vi "MGI Find 2D Intersection of 2 Lines.vi"(8 "error in (no error)":errorcluster, 10 "Line 2[start, end][x,y]":dbl[][](array[numeric]) format="%#.15f", 11 "Line 1[start, end][x,y]":dbl[][](array[numeric])) -> (0 "error out":errorcluster, 1 "Intersection within Line2 Segment?":bool, 2 "Intersection within Line1 Segment?":bool, 3 "Intersection[x,y]":dbl[](array[numeric]) format="%#_12g")   [LabVIEW 2016]
doc: "Finds the intersection of 2 lines. If the lines are parallel, then an argument error (code 1) is output.\nThe lines are specified using 2 points for each line. The points are specified as rows in a 2D array where the first column is x and the second is y.\n\nAuthored by Shawn D. Walpole\nsupport@mooregoodideas.com\nwww.mooregoodideas.com\n\nCopyright (c) 2010, Moore Good Ideas, Inc.\n\nAll rights reserved.\n\nRedistribution and use in source and binary forms, with or without modification, are permitted provided that the following conditions are met:\n\n * Redistributions of source code must retain the above copyright notice, this list of conditions and the following disclaimer.\n * Redistributions in binary form must reproduce the above copyright notice, this list of conditions and the following disclaimer in the documentation and/or other materials provided with the distribution.\n * Neither the name of Moore Good Ideas, Inc. nor the names of its contributors may be used to endorse or promote products derived from this software without specific prior written permission.\n\nTHIS SOFTWARE IS PROVIDED BY THE COPYRIGHT HOLDERS AND CONTRIBUTORS \"AS IS\" AND ANY EXPRESS OR IMPLIED WARRANTIES, INCLUDING, BUT NOT LIMITED TO, THE IMPLIED WARRANTIES OF MERCHANTABILITY AND FITNESS FOR A PARTICULAR PURPOSE ARE DISCLAIMED. IN NO EVENT SHALL THE COPYRIGHT OWNER OR CONTRIBUTORS BE LIABLE FOR ANY DIRECT, INDIRECT, INCIDENTAL, SPECIAL, EXEMPLARY, OR CONSEQUENTIAL DAMAGES (INCLUDING, BUT NOT LIMITED TO, PROCUREMENT OF SUBSTITUTE GOODS OR SERVICES; LOSS OF USE, DATA, OR PROFITS; OR BUSINESS INTERRUPTION) HOWEVER CAUSED AND ON ANY THEORY OF LIABILITY, WHETHER IN CONTRACT, STRICT LIABILITY, OR TORT (INCLUDING NEGLIGENCE OR OTHERWISE) ARISING IN ANY WAY OUT OF THE USE OF THIS SOFTWARE, EVEN IF ADVISED OF THE POSSIBILITY OF SUCH DAMAGE."
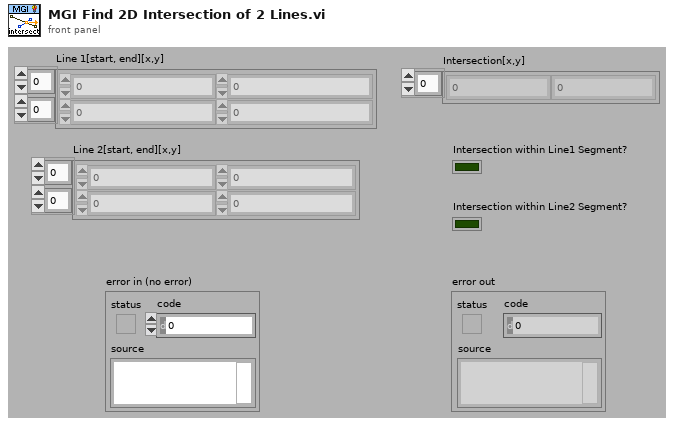
[diagram p1: front panel]
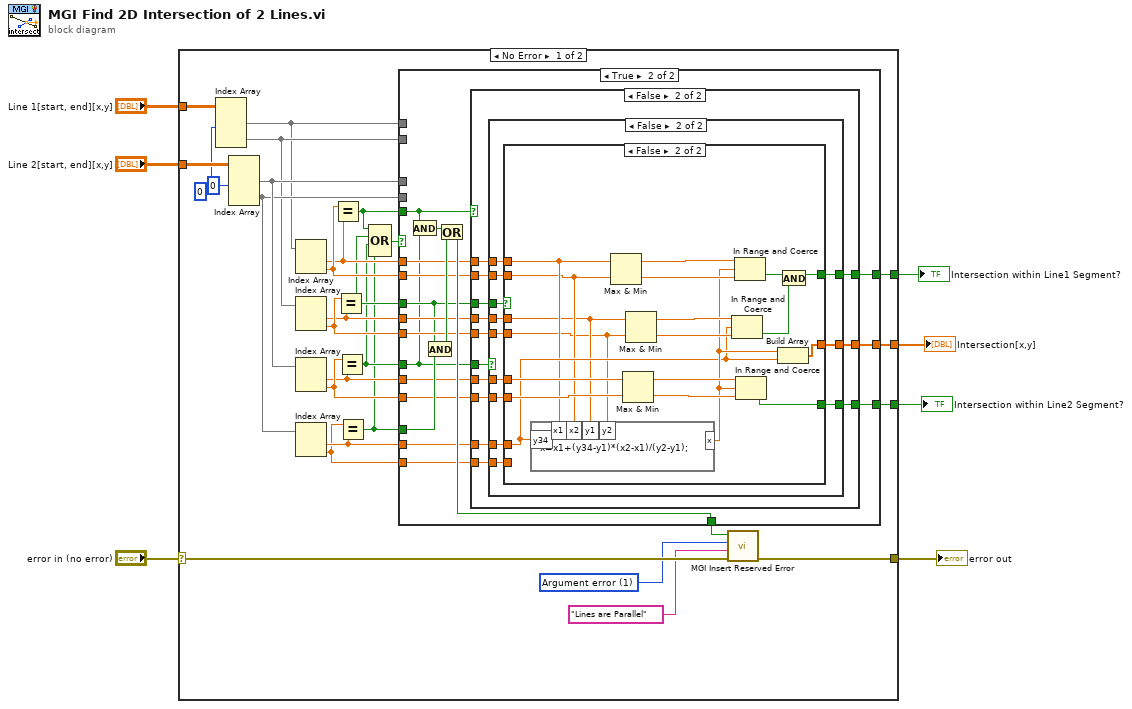
[diagram p0: block diagram]
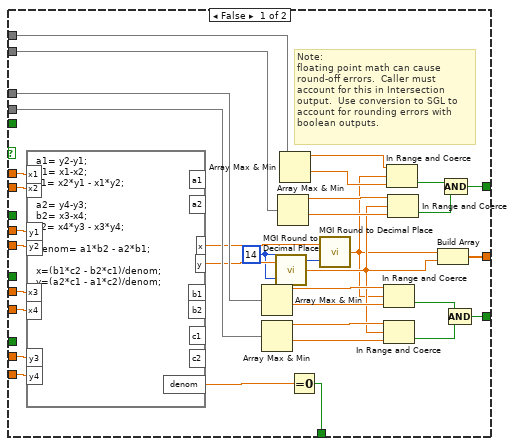
[diagram p2: hidden frame]
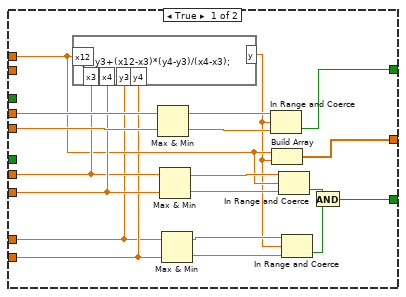
[diagram p3: hidden frame]
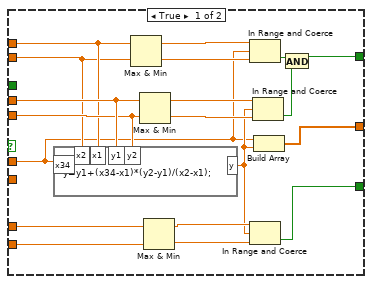
[diagram p4: hidden frame]
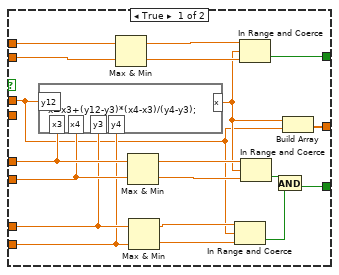
[diagram p5: hidden frame]
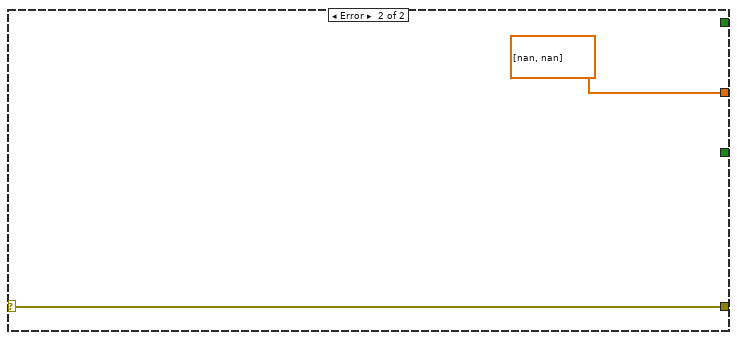
[diagram p6: hidden frame]
diagram:
  n1 = case shown="No Error" "error in (no error)" {
    selector: "error in (no error)" -> [w35 w191]
    tunnel: [w34 w191] -> w6
    tunnel: "Line 1[start, end][x,y]" -> [w30 _]
    tunnel: "Line 2[start, end][x,y]" -> [w29 _]
    tunnel: [w36 dbl[] [nan, nan]] -> w3
    tunnel: [w28 _] -> w2
    tunnel: [w27 _] -> w1
    frame No Error {
      w32 = u16 1 items=["No error", "Argument error", "Memory is full", "Out of zone", "End of file", "File already open", "Generic file I/O error", "File not found", "File permission error", "Disk is full", "Duplicate path", "Too many files open", "System feature not enabled", "Resource file not found", "Cannot add resource", "Resource not found", "Image not found", "Image memory error", "Pen does not exist", "Config type invalid", "Config token not found", "Config parse error", "Config memory error", "Bad external code format", "Bad external code offset", "External code not present", "Null window", "Destroy window error", "Null menu", "Print aborted", "Bad print record", "Print driver error", "Windows error during printing", "Memory error during printing", "Print dialog error", "Generic print error", "Invalid device refnum", "Device not found", "Device parameter error", "Device unit error", "Cannot open device", "Device call aborted", "Generic error", "Cancelled by user", "Object ID too low", "Object ID too high", "Object not in heap", "Unknown heap", "Unknown object (invalid DefProc)", "Unknown object (DefProc not in table)", "Message out of range", "Invalid (null) method", "Unknown message", "Manager call not supported", "Bad address", "Network operation in progress", "Network operation timed out", "Connection is busy", "Network attribute not supported", "Network error", "Address in use", "System out of memory", "Connection aborted", "Connection refused", "Not connected", "Already connected", "Connection closed", "Initialization error (interapplication manager)", "Bad occurrence", "Wait on unbound occurrence handler", "Occurrence queue overflow", "Datalog type conflict", "Unused", "Unrecognized type (interapplication manager)", "Memory corrupt", "Failed to make temporary DLL", "Old CIN version", "Drag socket not found", "Failed to load drop-object", "Failed to register OLE object", "Failed to release OLE object", "Format specifier type mismatch", "Unknown format specifier", "Too few format specifiers", "Too many format specifiers", "Scan failed", "Newer CIN version", "OLE Convert", "Runtime menu error", "Password tampered", "Unknown error code"] ("Reserved Error Code (Generic error)")
      n2 = Index Array(array=w30, index (col) #1=0 ("disabled index (col)")) -> (element #1=w21:dbl[], element #2=w22:dbl[])  [unwired: 3 in]
      n3 = Index Array(array=w29, index (col) #1=0 ("disabled index (col)")) -> (element #1=w24:dbl[], element #2=w23:dbl[])  [unwired: 3 in]
      n4 = Index Array(array=w21) -> (element #1=w19:dbl, element #2=w20:dbl)  [unwired: 2 in]
      n5 = Index Array(array=w22) -> (element #1=w17:dbl, element #2=w18:dbl)  [unwired: 2 in]
      n6 = Index Array(array=w24) -> (element #1=w15:dbl, element #2=w16:dbl)  [unwired: 2 in]
      n7 = Index Array(array=w23) -> (element #1=w14:dbl, element #2=w13:dbl)  [unwired: 2 in]
      n8 = Equal?(x=w20, y=w19) -> (x = y?=w11:bool)
      n9 = Equal?(x=w18, y=w17) -> (x = y?=w10:bool)
      n10 = Equal?(x=w16, y=w15) -> (x = y?=w9:bool)
      n11 = Equal?(x=w13, y=w14) -> (x = y?=w8:bool)
      n12 = Compound Arithmetic op=OR(w11, w10, w9, w8) -> (w12:bool)
      n13 = case shown="True" w12 {
        tunnel: [w70 w75] -> w36
        tunnel: [w68 w85] -> w33
        tunnel: [w63 w74] -> w28
        tunnel: [w62 w73] -> w27
        tunnel: w24 -> [w53 _]
        tunnel: w23 -> [w52 _]
        tunnel: w22 -> [w51 _]
        tunnel: w21 -> [w50 _]
        tunnel: w20 -> [w44 w82]
        tunnel: w19 -> [w43 w83]
        tunnel: w18 -> [w42 w80]
        tunnel: w17 -> [w41 w81]
        tunnel: w16 -> [w40 w78]
        tunnel: w15 -> [w39 w79]
        tunnel: w14 -> [w38 w77]
        tunnel: w13 -> [w37 w76]
        tunnel: w11 -> [_ w84]
        tunnel: w10 -> [_ w72]
        tunnel: w9 -> [_ w71]
        tunnel: w8 -> [_ w88]
        frame False {
          w45 = 14 ("Decimal Digits")
          # "Note:\nfloating point math can cause round-off errors.  Caller must account for this in Intersection output.  Use conversion to SGL to account for rounding errors with boolean outputs."
          n14 = formula code="a1= y2-y1;\nb1= x1-x2;\nc1= x2*y1 - x1*y2;\n\na2= y4-y3;\nb2= x3-x4;\nc2= x4*y3 - x3*y4;\n\ndenom= a1*b2 - a2*b1;\n\nx=(b1*c2 - b2*c1)/denom;\ny=(a2*c1 - a1*c2)/denom;"("y2"=w42, "y1"=w41, "x2"=w44, "x1"=w43, "y4"=w37, "y3"=w38, "x4"=w40, "x3"=w39) -> ("denom"=w69:dbl, "x"=w47:dbl, "y"=w49:dbl)  [unwired: 6 out]
          n15 = Array Max & Min(array=w53) -> (max value=w57:dbl, min value=w56:dbl)  [unwired: 2 out]
          n16 = Array Max & Min(array=w52) -> (max value=w55:dbl, min value=w54:dbl)  [unwired: 2 out]
          n17 = call <userlib>:"MGI Round to Decimal Place.vi"("Decimal Digits"=w45, "Number"=w49) -> ("Rounded"=w48:dbl)  [unwired: 1 in]
          n18 = Array Max & Min(array=w51) -> (max value=w59:dbl, min value=w58:dbl)  [unwired: 2 out]
          n19 = Array Max & Min(array=w50) -> (max value=w61:dbl, min value=w60:dbl)  [unwired: 2 out]
          n20 = Equal To 0?(x=w69) -> (x = 0?=w68:bool)
          n21 = call <userlib>:"MGI Round to Decimal Place.vi"("Decimal Digits"=w45, "Number"=w47) -> ("Rounded"=w46:dbl)  [unwired: 1 in]
          n22 = In Range and Coerce(upper limit=w57, x=w46, lower limit=w56) -> (In Range?=w67:bool)  [unwired: 1 out]
          n23 = In Range and Coerce(upper limit=w55, x=w48, lower limit=w54) -> (In Range?=w66:bool)  [unwired: 1 out]
          n24 = In Range and Coerce(upper limit=w61, x=w46, lower limit=w60) -> (In Range?=w65:bool)  [unwired: 1 out]
          n25 = In Range and Coerce(upper limit=w59, x=w48, lower limit=w58) -> (In Range?=w64:bool)  [unwired: 1 out]
          n26 = Build Array(w46, w48) -> (w70:dbl[])
          n27 = Compound Arithmetic op=AND(w65, w64) -> (w63:bool)
          n28 = Compound Arithmetic op=AND(w67, w66) -> (w62:bool)
        }
        frame True {
          n29 = And(x=w84, y=w71) -> (x .and. y?=w86:bool)
          n30 = And(x=w72, y=w88) -> (x .and. y?=w87:bool)
          n31 = Or(x=w86, y=w87) -> (x .or. y?=w85:bool)
          n32 = case shown="False" w84 {
            tunnel: w83 -> [w97 w114]
            tunnel: w82 -> [_ w108]
            tunnel: w81 -> [w104 w117]
            tunnel: w80 -> [w105 w118]
            tunnel: w79 -> [w100 w115]
            tunnel: w78 -> [w101 w116]
            tunnel: w77 -> [w95 w112]
            tunnel: w76 -> [w96 w113]
            tunnel: [w107 w120] -> w75
            tunnel: [w106 w119] -> w74
            tunnel: [w89 w111] -> w73
            tunnel: w72 -> [_ w109]
            tunnel: w71 -> [_ w110]
            frame True {
              n33 = formula code="y=y3+(x12-x3)*(y4-y3)/(x4-x3);"("x12"=w97, "x3"=w100, "x4"=w101, "y3"=w95, "y4"=w96) -> ("y"=w92:dbl)
              n34 = Max & Min(x=w104, y=w105) -> (max(x,y)=w103:dbl, min(x,y)=w102:dbl)
              n35 = Max & Min(x=w100, y=w101) -> (max(x,y)=w99:dbl, min(x,y)=w98:dbl)
              n36 = Max & Min(x=w95, y=w96) -> (max(x,y)=w93:dbl, min(x,y)=w94:dbl)
              n37 = In Range and Coerce(upper limit=w103, x=w92, lower limit=w102) -> (In Range?=w106:bool)  [unwired: 1 out]
              n38 = Build Array(w97, w92) -> (w107:dbl[])
              n39 = In Range and Coerce(upper limit=w99, x=w97, lower limit=w98) -> (In Range?=w90:bool)  [unwired: 1 out]
              n40 = In Range and Coerce(upper limit=w93, x=w92, lower limit=w94) -> (In Range?=w91:bool)  [unwired: 1 out]
              n41 = And(x=w90, y=w91) -> (x .and. y?=w89:bool)
            }
            frame False {
              n42 = case shown="False" w110 {
                tunnel: [w139 w151] -> w120
                tunnel: [w123 w143] -> w119
                tunnel: w118 -> [w127 w147]
                tunnel: w117 -> [w128 w148]
                tunnel: w116 -> [_ w140]
                tunnel: w115 -> [w121 w142]
                tunnel: w114 -> [w125 w145]
                tunnel: w113 -> [w133 w150]
                tunnel: w112 -> [w132 w149]
                tunnel: [w126 w146] -> w111
                tunnel: w109 -> [_ w141]
                tunnel: w108 -> [w124 w144]
                frame True {
                  n43 = formula code="y=y1+(x34-x1)*(y2-y1)/(x2-x1);"("x1"=w125, "x34"=w121, "x2"=w124, "y1"=w128, "y2"=w127) -> ("y"=w129:dbl)
                  n44 = Max & Min(x=w125, y=w124) -> (max(x,y)=w135:dbl, min(x,y)=w134:dbl)
                  n45 = Max & Min(x=w128, y=w127) -> (max(x,y)=w137:dbl, min(x,y)=w136:dbl)
                  n46 = Max & Min(x=w132, y=w133) -> (max(x,y)=w130:dbl, min(x,y)=w131:dbl)
                  n47 = In Range and Coerce(upper limit=w135, x=w121, lower limit=w134) -> (In Range?=w122:bool)  [unwired: 1 out]
                  n48 = In Range and Coerce(upper limit=w130, x=w129, lower limit=w131) -> (In Range?=w126:bool)  [unwired: 1 out]
                  n49 = In Range and Coerce(upper limit=w137, x=w129, lower limit=w136) -> (In Range?=w138:bool)  [unwired: 1 out]
                  n50 = Build Array(w121, w129) -> (w139:dbl[])
                  n51 = And(x=w122, y=w138) -> (x .and. y?=w123:bool)
                }
                frame False {
                  n52 = case shown="False" w141 {
                    tunnel: [w170 w189] -> w151
                    tunnel: w150 -> [w157 _]
                    tunnel: w149 -> [w158 w179]
                    tunnel: w148 -> [w154 w176]
                    tunnel: w147 -> [_ w175]
                    tunnel: [w153 w174] -> w146
                    tunnel: w145 -> [w162 w178]
                    tunnel: w144 -> [w161 w177]
                    tunnel: [w155 w171] -> w143
                    tunnel: w142 -> [w160 w182]
                    tunnel: w140 -> [w159 w181]
                    frame True {
                      n53 = formula code="x=x3+(y12-y3)*(x4-x3)/(y4-y3);"("y3"=w158, "y12"=w154, "y4"=w157, "x3"=w160, "x4"=w159) -> ("x"=w156:dbl)
                      n54 = Max & Min(x=w162, y=w161) -> (max(x,y)=w167:dbl, min(x,y)=w166:dbl)
                      n55 = Max & Min(x=w160, y=w159) -> (max(x,y)=w169:dbl, min(x,y)=w168:dbl)
                      n56 = Max & Min(x=w158, y=w157) -> (max(x,y)=w164:dbl, min(x,y)=w165:dbl)
                      n57 = In Range and Coerce(upper limit=w164, x=w154, lower limit=w165) -> (In Range?=w163:bool)  [unwired: 1 out]
                      n58 = In Range and Coerce(upper limit=w167, x=w156, lower limit=w166) -> (In Range?=w155:bool)  [unwired: 1 out]
                      n59 = In Range and Coerce(upper limit=w169, x=w156, lower limit=w168) -> (In Range?=w152:bool)  [unwired: 1 out]
                      n60 = And(x=w152, y=w163) -> (x .and. y?=w153:bool)
                      n61 = Build Array(w156, w154) -> (w170:dbl[])
                    }
                    frame False {
                      n62 = formula code="x=x1+(y34-y1)*(x2-x1)/(y2-y1);"("y1"=w176, "y34"=w179, "y2"=w175, "x1"=w178, "x2"=w177) -> ("x"=w180:dbl)
                      n63 = Max & Min(x=w178, y=w177) -> (max(x,y)=w186:dbl, min(x,y)=w185:dbl)
                      n64 = Max & Min(x=w182, y=w181) -> (max(x,y)=w188:dbl, min(x,y)=w187:dbl)
                      n65 = Max & Min(x=w176, y=w175) -> (max(x,y)=w183:dbl, min(x,y)=w184:dbl)
                      n66 = In Range and Coerce(upper limit=w183, x=w179, lower limit=w184) -> (In Range?=w173:bool)  [unwired: 1 out]
                      n67 = In Range and Coerce(upper limit=w186, x=w180, lower limit=w185) -> (In Range?=w172:bool)  [unwired: 1 out]
                      n68 = In Range and Coerce(upper limit=w188, x=w180, lower limit=w187) -> (In Range?=w174:bool)  [unwired: 1 out]
                      n69 = Build Array(w180, w179) -> (w189:dbl[])
                      n70 = And(x=w172, y=w173) -> (x .and. y?=w171:bool)
                    }
                  }
                }
              }
            }
          }
        }
      }
      n71 = call <userlib>:"MGI Insert Reserved Error.vi"("Error In"=w35, "Error Description"="Lines are Parallel" ("error description"), "Reserved Error Code (Generic error)"=w32, "Error? (T)"=w33) -> ("Error Out"=w34:errorcluster)  [unwired: 7 in]
    }
    frame Error {
    }
  }
  "error out" <- w6
  "Intersection[x,y]" <- w3
  "Intersection within Line2 Segment?" <- w1
  "Intersection within Line1 Segment?" <- w2
